vi "Format CSV.vi"(8 "error in (no error)":errorcluster, 9 "delimiter":string=",", 10 "CSV File Input":path, 11 "Original CSV Format":enum16{"Format A", "Format B"}(ring)) -> (0 "error out":errorcluster, 1 "Parcel Length":i32[](array[numeric]), 2 "All Terminal Data":T1(array[cluster]))   [LabVIEW 2017] (continued)
"22:36.1", "22:36.1", "22:36.2", "22:36.2", "22:36.2", "22:36.3", "22:36.3", "22:36.3", "22:36.4", "22:36.4", "22:36.4", "22:36.5", "22:36.5", "22:36.5", "22:36.6", "22:36.6", "22:36.6", "22:36.7", "22:36.7", "22:36.7", "22:36.8", "22:36.8", "22:36.8", "22:36.9", "22:36.9", "22:36.9", "22:37.0", "22:37.0", "22:37.0", "22:37.1", "22:37.1", "22:37.1", "22:37.2", "22:37.2", "22:37.2", "22:37.3", "22:37.3", "22:37.3", "22:37.4", "22:37.4", "22:37.4", "22:37.5", "22:37.5", "22:37.5", "22:37.6", "22:37.6", "22:37.6", "22:37.7", "22:37.7", "22:37.7", "22:37.8", "22:37.8", "22:37.8", "22:37.9", "22:37.9", "22:37.9", "22:38.0", "22:38.0", "22:38.0", "22:38.1", "22:38.1", "22:38.1", "22:38.2", "22:38.2", "22:38.2", "22:38.3", "22:38.3", "22:38.3", "22:38.4", "22:38.4", "22:38.4", "22:38.5", "22:38.5", "22:38.5", "22:38.6", "22:38.6", "22:38.6", "22:38.7", "22:38.7", "22:38.7", "22:38.8", "22:38.8", "22:38.8", "22:38.9", "22:38.9", "22:38.9", "22:39.0", "22:39.0", "22:39.0", "22:39.1", "22:39.1", "22:39.1", "22:39.2", "22:39.2", "22:39.2", "22:39.3", "22:39.3", "22:39.3", "22:39.4", "22:39.4", "22:39.4", "22:39.5", "22:39.5", "22:39.5", "22:39.6", "22:39.6", "22:39.6", "22:39.7", "22:39.7", "22:39.7", "22:39.8", "22:39.8", "22:39.8", "22:39.9", "22:39.9", "22:39.9", "22:40.0", "22:40.0", "22:40.0", "22:40.1", "22:40.1", "22:40.1", "22:40.2", "22:40.2", "22:40.2", "22:40.3", "22:40.3", "22:40.3", "22:40.4", "22:40.4", "22:40.4", "22:40.5", "22:40.5", "22:40.5", "22:40.6", "22:40.6", "22:40.6", "22:40.7", "22:40.7", "22:40.7", "22:40.8", "22:40.8", "22:40.8", "22:40.9", "22:40.9", "22:40.9", "22:41.0", "22:41.0", "22:41.0", "22:41.1", "22:41.1", "22:41.1", "22:41.2", "22:41.2", "22:41.2", "22:41.3", "22:41.3", "22:41.3", "22:41.4", "22:41.4", "22:41.4", "22:41.5", "22:41.5", "22:41.5", "22:41.6", "22:41.6", "22:41.6", "22:41.7", "22:41.7", "22:41.7", "22:41.8", "22:41.8", "22:41.8", "22:41.9", "22:41.9", "22:41.9", "22:42.0", "22:42.0", "22:42.0", "22:42.1", "22:42.1", "22:42.1", "22:42.2", "22:42.2", "22:42.2", "22:42.3", "22:42.3", "22:42.3", "22:42.4", "22:42.4", "22:42.4", "22:42.5", "22:42.5", "22:42.5", "22:42.6", "22:42.6", "22:42.6", "22:42.7", "22:42.7", "22:42.7", "22:42.8", "22:42.8", "22:42.8", "22:42.9", "22:42.9", "22:42.9", "22:43.0", "22:43.0", "22:43.0", "22:43.1", "22:43.1", "22:43.1", "22:43.2", "22:43.2", "22:43.2", "22:43.3", "22:43.3", "22:43.3", "22:43.4", "22:43.4", "22:43.4", "22:43.5", "22:43.5", "22:43.5", "22:43.6", "22:43.6", "22:43.6", "22:43.7", "22:43.7", "22:43.7", "22:43.8", "22:43.8", "22:43.8", "22:43.9", "22:43.9", "22:43.9", "22:44.0", "22:44.0", "22:44.0", "22:44.1", "22:44.1", "22:44.1", "22:44.2", "22:44.2", "22:44.2", "22:44.3", "22:44.3", "22:44.3", "22:44.4", "22:44.4", "22:44.4", "22:44.5", "22:44.5", "22:44.5", "22:44.6", "22:44.6", "22:44.6", "22:44.7", "22:44.7", "22:44.7", "22:44.8", "22:44.8", "22:44.8", "22:44.9", "22:44.9", "22:44.9", "22:45.0", "22:45.0", "22:45.0", "22:45.1", "22:45.1", "22:45.1", "22:45.2", "22:45.2", "22:45.2", "22:45.3", "22:45.3", "22:45.3", "22:45.4", "22:45.4", "22:45.4", "22:45.5", "22:45.5", "22:45.5", "22:45.6", "22:45.6", "22:45.6", "22:45.7", "22:45.7", "22:45.7", "22:45.8", "22:45.8", "22:45.8", "22:45.9", "22:45.9", "22:45.9", "22:46.0", "22:46.0", "22:46.0", "22:46.1", "22:46.1", "22:46.1", "22:46.2", "22:46.2", "22:46.2", "22:46.3", "22:46.3", "22:46.3", "22:46.4", "22:46.4", "22:46.4", "22:46.5", "22:46.5", "22:46.5", "22:46.6", "22:46.6", "22:46.6", "22:46.7", "22:46.7", "22:46.7", "22:46.8", "22:46.8", "22:46.8", "22:46.9", "22:46.9", "22:46.9", "22:47.0", "22:47.0", "22:47.0", "22:47.1", "22:47.1", "22:47.1", "22:47.2", "22:47.2", "22:47.2", "22:47.3", "22:47.3", "22:47.3", "22:47.4", "22:47.4", "22:47.4", "22:47.5", "22:47.5", "22:47.5", "22:47.6", "22:47.6", "22:47.6", "22:47.7", "22:47.7", "22:47.7", "22:47.8", "22:47.8", "22:47.8", "22:47.9", "22:47.9", "22:47.9", "22:48.0", "22:48.0", "22:48.0", "22:48.1", "22:48.1", "22:48.1", "22:48.2", "22:48.2", "22:48.2", "22:48.3", "22:48.3", "22:48.3", "22:48.4", "22:48.4", "22:48.4", "22:48.5", "22:48.5", "22:48.5", "22:48.6", "22:48.6", "22:48.6", "22:48.7", "22:48.7", "22:48.7", "22:48.8", "22:48.8", "22:48.8", "22:48.9", "22:48.9", "22:48.9", "22:49.0", "22:49.0", "22:49.0", "22:49.1", "22:49.1", "22:49.1", "22:49.2", "22:49.2", "22:49.2", "22:49.3", "22:49.3", "22:49.3", "22:49.4", "22:49.4", "22:49.4", "22:49.5", "22:49.5", "22:49.5", "22:49.6", "22:49.6", "22:49.6", "22:49.7", "22:49.7", "22:49.7", "22:49.8", "22:49.8", "22:49.8", "22:49.9", "22:49.9", "22:49.9", "22:50.0", "22:50.0", "22:50.0", "22:50.1", "22:50.1", "22:50.1", "22:50.2", "22:50.2", "22:50.2", "22:50.3", "22:50.3", "22:50.3", "22:50.4", "22:50.4", "22:50.4", "22:50.5", "22:50.5", "22:50.5", "22:50.6", "22:50.6", "22:50.6", "22:50.7", "22:50.7", "22:50.7", "22:50.8", "22:50.8", "22:50.8", "22:50.9", "22:50.9", "22:50.9", "22:51.0", "22:51.0", "22:51.0", "22:51.1", "22:51.1", "22:51.1", "22:51.2", "22:51.2", "22:51.2", "22:51.3", "22:51.3", "22:51.3", "22:51.4", "22:51.4", "22:51.4", "22:51.5", "22:51.5", "22:51.5", "22:51.6", "22:51.6", "22:51.6", "22:51.7", "22:51.7", "22:51.7", "22:51.8", "22:51.8", "22:51.8", "22:51.9", "22:51.9", "22:51.9", "22:52.0", "22:52.0", "22:52.0", "22:52.1", "22:52.1", "22:52.1", "22:52.2", "22:52.2", "22:52.2", "22:52.3", "22:52.3", "22:52.3", "22:52.4", "22:52.4", "22:52.4", "22:52.5", "22:52.5", "22:52.5", "22:52.6", "22:52.6", "22:52.6", "22:52.7", "22:52.7", "22:52.7", "22:52.8", "22:52.8", "22:52.8", "22:52.9", "22:52.9", "22:52.9", "22:53.0", "22:53.0", "22:53.0", "22:53.1", "22:53.1", "22:53.1", "22:53.2", "22:53.2", "22:53.2", "22:53.3", "22:53.3", "22:53.3", "22:53.4", "22:53.4", "22:53.4", "22:53.5", "22:53.5", "22:53.5", "22:53.6", "22:53.6", "22:53.6", "22:53.7", "22:53.7", "22:53.7", "22:53.8", "22:53.8", "22:53.8", "22:53.9", "22:53.9", "22:53.9", "22:54.0", "22:54.0", "22:54.0", "22:54.1", "22:54.1", "22:54.1", "22:54.2", "22:54.2", "22:54.2", "22:54.3", "22:54.3", "22:54.3", "22:54.4", "22:54.4", "22:54.4", "22:54.5", "22:54.5", "22:54.5", "22:54.6", "22:54.6", "22:54.6", "22:54.7", "22:54.7", "22:54.7", "22:54.8", "22:54.8", "22:54.8", "22:54.9", "22:54.9", "22:54.9", "22:55.0", "22:55.0", "22:55.0", "22:55.1", "22:55.1", "22:55.1", "22:55.2", "22:55.2", "22:55.2", "22:55.3", "22:55.3", "22:55.3", "22:55.4", "22:55.4", "22:55.4", "22:55.5", "22:55.5", "22:55.5", "22:55.6", "22:55.6", "22:55.6", "22:55.7", "22:55.7", "22:55.7", "22:55.8", "22:55.8", "22:55.8", "22:55.9", "22:55.9", "22:55.9", "22:56.0", "22:56.0", "22:56.0", "22:56.1", "22:56.1", "22:56.1", "22:56.2", "22:56.2", "22:56.2", "22:56.3", "22:56.3", "22:56.3", "22:56.4", "22:56.4", "22:56.4", "22:56.5", "22:56.5", "22:56.5", "22:56.6", "22:56.6", "22:56.6", "22:56.7", "22:56.7", "22:56.7", "22:56.8", "22:56.8", "22:56.8", "22:56.9", "22:56.9", "22:56.9", "22:57.0", "22:57.0", "22:57.0", "22:57.1", "22:57.1", "22:57.1", "22:57.2", "22:57.2", "22:57.2", "22:57.3", "22:57.3", "22:57.3", "22:57.4", "22:57.4", "22:57.4", "22:57.5", "22:57.5", "22:57.5", "22:57.6", "22:57.6", "22:57.6", "22:57.7", "22:57.7", "22:57.7", "22:57.8", "22:57.8", "22:57.8", "22:57.9", "22:57.9", "22:57.9", "22:58.0", "22:58.0", "22:58.0", "22:58.1", "22:58.1", "22:58.1", "22:58.2", "22:58.2", "22:58.2", "22:58.3", "22:58.3", "22:58.3", "22:58.4", "22:58.4", "22:58.4", "22:58.5", "22:58.5", "22:58.5", "22:58.6", "22:58.6", "22:58.6", "22:58.7", "22:58.7", "22:58.7", "22:58.8", "22:58.8", "22:58.8", "22:58.9", "22:58.9", "22:58.9", "22:59.0", "22:59.0", "22:59.0", "22:59.1", "22:59.1", "22:59.1", "22:59.2", "22:59.2", "22:59.2", "22:59.3", "22:59.3", "22:59.3", "22:59.4", "22:59.4", "22:59.4", "22:59.5", "22:59.5", "22:59.5", "22:59.6", "22:59.6", "22:59.6", "22:59.7", "22:59.7", "22:59.7", "22:59.8", "22:59.8", "22:59.8", "22:59.9", "22:59.9", "22:59.9", "23:00.0", "23:00.0", "23:00.0", "23:00.1", "23:00.1", "23:00.1", "23:00.2", "23:00.2", "23:00.2", "23:00.3", "23:00.3", "23:00.3", "23:00.4", "23:00.4", "23:00.4", "23:00.5", "23:00.5", "23:00.5", "23:00.6", "23:00.6", "23:00.6", "23:00.7", "23:00.7", "23:00.7", "23:00.8", "23:00.8", "23:00.8", "23:00.9", "23:00.9", "23:00.9", "23:01.0", "23:01.0", "23:01.0", "23:01.1", "23:01.1", "23:01.1", "23:01.2", "23:01.2", "23:01.2", "23:01.3", "23:01.3", "23:01.3", "23:01.4", "23:01.4", "23:01.4", "23:01.5", "23:01.5", "23:01.5", "23:01.6", "23:01.6", "23:01.6", "23:01.7", "23:01.7", "23:01.7", "23:01.8", "23:01.8", "23:01.8", "23:01.9", "23:01.9", "23:01.9", "23:02.0", "23:02.0", "23:02.0", "23:02.1", "23:02.1", "23:02.1", "23:02.2", "23:02.2", "23:02.2", "23:02.3", "23:02.3", "23:02.3", "23:02.4", "23:02.4", "23:02.4", "23:02.5", "23:02.5", "23:02.5", "23:02.6", "23:02.6", "23:02.6", "23:02.7", "23:02.7", "23:02.7", "23:02.8", "23:02.8", "23:02.8", "23:02.9", "23:02.9", "23:02.9", "23:03.0", "23:03.0", "23:03.0", "23:03.1", "23:03.1", "23:03.1", "23:03.2", "23:03.2", "23:03.2", "23:03.3", "23:03.3", "23:03.3", "23:03.4", "23:03.4", "23:03.4", "23:03.5", "23:03.5", "23:03.5", "23:03.6", "23:03.6", "23:03.6", "23:03.7", "23:03.7", "23:03.7", "23:03.8", "23:03.8", "23:03.8", "23:03.9", "23:03.9", "23:03.9", "23:04.0", "23:04.0", "23:04.0", "23:04.1", "23:04.1", "23:04.1", "23:04.2", "23:04.2", "23:04.2", "23:04.3", "23:04.3", "23:04.3", "23:04.4", "23:04.4", "23:04.4", "23:04.5", "23:04.5", "23:04.5", "23:04.6", "23:04.6", "23:04.6", "23:04.7", "23:04.7", "23:04.7", "23:04.8", "23:04.8", "23:04.8", "23:04.9", "23:04.9", "23:04.9", "23:05.0", "23:05.0", "23:05.0", "23:05.1", "23:05.1", "23:05.1", "23:05.2", "23:05.2", "23:05.2", "23:05.3", "23:05.3", "23:05.3", "23:05.4", "23:05.4", "23:05.4", "23:05.5", "23:05.5", "23:05.5", "23:05.6", "23:05.6", "23:05.6", "23:05.7", "23:05.7", "23:05.7", "23:05.8", "23:05.8", "23:05.8", "23:05.9", "23:05.9", "23:05.9", "23:06.0", "23:06.0", "23:06.0", "23:06.1", "23:06.1", "23:06.1", "23:06.2", "23:06.2", "23:06.2", "23:06.3", "23:06.3", "23:06.3", "23:06.4", "23:06.4", "23:06.4", "23:06.5", "23:06.5", "23:06.5", "23:06.6", "23:06.6", "23:06.6", "23:06.7", "23:06.7", "23:06.7", "23:06.8", "23:06.8", "23:06.8", "23:06.9", "23:06.9", "23:06.9", "23:07.0", "23:07.0", "23:07.0", "23:07.1", "23:07.1", "23:07.1", "23:07.2", "23:07.2", "23:07.2", "23:07.3", "23:07.3", "23:07.3", "23:07.4", "23:07.4", "23:07.4", "23:07.5", "23:07.5", "23:07.5", "23:07.6", "23:07.6", "23:07.6", "23:07.7", "23:07.7", "23:07.7", "23:07.8", "23:07.8", "23:07.8", "23:07.9", "23:07.9", "23:07.9", "23:08.0", "23:08.0", "23:08.0", "23:08.1", "23:08.1", "23:08.1", "23:08.2", "23:08.2", "23:08.2", "23:08.3", "23:08.3", "23:08.3", "23:08.4", "23:08.4", "23:08.4", "23:08.5", "23:08.5", "23:08.5", "23:08.6", "23:08.6", "23:08.6", "23:08.7", "23:08.7", "23:08.7", "23:08.8", "23:08.8", "23:08.8", "23:08.9", "23:08.9", "23:08.9", "23:09.0", "23:09.0", "23:09.0", "23:09.1", "23:09.1", "23:09.1", "23:09.2", "23:09.2", "23:09.2", "23:09.3", "23:09.3", "23:09.3", "23:09.4", "23:09.4", "23:09.4", "23:09.5", "23:09.5", "23:09.5", "23:09.6", "23:09.6", "23:09.6", "23:09.7", "23:09.7", "23:09.7", "23:09.8", "23:09.8", "23:09.8", "23:09.9", "23:09.9", "23:09.9", "23:10.0", "23:10.0", "23:10.0", "23:10.1", "23:10.1", "23:10.1", "23:10.2", "23:10.2", "23:10.2", "23:10.3", "23:10.3", "23:10.3", "23:10.4", "23:10.4", "23:10.4", "23:10.5", "23:10.5", "23:10.5", "23:10.6", "23:10.6", "23:10.6", "23:10.7", "23:10.7", "23:10.7", "23:10.8", "23:10.8", "23:10.8", "23:10.9", "23:10.9", "23:10.9", "23:11.0", "23:11.0", "23:11.0", "23:11.1", "23:11.1", "23:11.1", "23:11.2", "23:11.2", "23:11.2", "23:11.3", "23:11.3", "23:11.3", "23:11.4", "23:11.4", "23:11.4", "23:11.5", "23:11.5", "23:11.5", "23:11.6", "23:11.6", "23:11.6", "23:11.7", "23:11.7", "23:11.7", "23:11.8", "23:11.8", "23:11.8", "23:11.9", "23:11.9", "23:11.9", "23:12.0", "23:12.0", "23:12.0", "23:12.1", "23:12.1", "23:12.1", "23:12.2", "23:12.2", "23:12.2", "23:12.3", "23:12.3", "23:12.3", "23:12.4", "23:12.4", "23:12.4", "23:12.5", "23:12.5", "23:12.5", "23:12.6", "23:12.6", "23:12.6", "23:12.7", "23:12.7", "23:12.7", "23:12.8", "23:12.8", "23:12.8", "23:12.9", "23:12.9", "23:12.9", "23:13.0", "23:13.0", "23:13.0", "23:13.1", "23:13.1", "23:13.1", "23:13.2", "23:13.2", "23:13.2", "23:13.3", "23:13.3", "23:13.3", "23:13.4", "23:13.4", "23:13.4", "23:13.5", "23:13.5", "23:13.5", "23:13.6", "23:13.6", "23:13.6", "23:13.7", "23:13.7", "23:13.7", "23:13.8", "23:13.8", "23:13.8", "23:13.9", "23:13.9", "23:13.9", "23:14.0", "23:14.0", "23:14.0", "23:14.1", "23:14.1", "23:14.1", "23:14.2", "23:14.2", "23:14.2", "23:14.3", "23:14.3", "23:14.3", "23:14.4", "23:14.4", "23:14.4", "23:14.5", "23:14.5", "23:14.5", "23:14.6", "23:14.6", "23:14.6", "23:14.7", "23:14.7", "23:14.7", "23:14.8", "23:14.8", "23:14.8", "23:14.9", "23:14.9", "23:14.9", "23:15.0", "23:15.0", "23:15.0", "23:15.1", "23:15.1", "23:15.1", "23:15.2", "23:15.2", "23:15.2", "23:15.3", "23:15.3", "23:15.3", "23:15.4", "23:15.4", "23:15.4", "23:15.5", "23:15.5", "23:15.5", "23:15.6", "23:15.6", "23:15.6", "23:15.7", "23:15.7", "23:15.7", "23:15.8", "23:15.8", "23:15.8", "23:15.9", "23:15.9", "23:15.9", "23:16.0", "23:16.0", "23:16.0", "23:16.1", "23:16.1", "23:16.1", "23:16.2", "23:16.2", "23:16.2", "23:16.3", "23:16.3", "23:16.3", "23:16.4", "23:16.4", "23:16.4", "23:16.5", "23:16.5", "23:16.5", "23:16.6", "23:16.6", "23:16.6", "23:16.7", "23:16.7", "23:16.7", "23:16.8", "23:16.8", "23:16.8", "23:16.9", "23:16.9", "23:16.9", "23:17.0", "23:17.0", "23:17.0", "23:17.1", "23:17.1", "23:17.1", "23:17.2", "23:17.2", "23:17.2", "23:17.3", "23:17.3", "23:17.3", "23:17.4", "23:17.4", "23:17.4", "23:17.5", "23:17.5", "23:17.5", "23:17.6", "23:17.6", "23:17.6", "23:17.7", "23:17.7", "23:17.7", "23:17.8", "23:17.8", "23:17.8", "23:17.9", "23:17.9", "23:17.9", "23:18.0", "23:18.0", "23:18.0", "23:18.1", "23:18.1", "23:18.1", "23:18.2", "23:18.2", "23:18.2", "23:18.3", "23:18.3", "23:18.3", "23:18.4", "23:18.4", "23:18.4", "23:18.5", "23:18.5", "23:18.5", "23:18.6", "23:18.6", "23:18.6", "23:18.7", "23:18.7", "23:18.7", "23:18.8", "23:18.8", "23:18.8", "23:18.9", "23:18.9", "23:18.9", "23:19.0", "23:19.0", "23:19.0", "23:19.1", "23:19.1", "23:19.1", "23:19.2", "23:19.2", "23:19.2", "23:19.3", "23:19.3", "23:19.3", "23:19.4", "23:19.4", "23:19.4", "23:19.5", "23:19.5", "23:19.5", "23:19.6", "23:19.6", "23:19.6", "23:19.7", "23:19.7", "23:19.7", "23:19.8", "23:19.8", "23:19.8", "23:19.9", "23:19.9", "23:19.9", "23:20.0", "23:20.0", "23:20.0", "23:20.1", "23:20.1", "23:20.1", "23:20.2", "23:20.2", "23:20.2", "23:20.3", "23:20.3", "23:20.3", "23:20.4", "23:20.4", "23:20.4", "23:20.5", "23:20.5", "23:20.5", "23:20.6", "23:20.6", "23:20.6", "23:20.7", "23:20.7", "23:20.7", "23:20.8", "23:20.8", "23:20.8", "23:20.9", "23:20.9", "23:20.9", "23:21.0", "23:21.0", "23:21.0", "23:21.1", "23:21.1", "23:21.1", "23:21.2", "23:21.2", "23:21.2", "23:21.3", "23:21.3", "23:21.3", "23:21.4", "23:21.4", "23:21.4", "23:21.5", "23:21.5", "23:21.5", "23:21.6", "23:21.6", "23:21.6", "23:21.7", "23:21.7", "23:21.7", "23:21.8", "23:21.8", "23:21.8", "23:21.9", "23:21.9", "23:21.9", "23:22.0", "23:22.0", "23:22.0", "23:22.1", "23:22.1", "23:22.1", "23:22.2", "23:22.2", "23:22.2", "23:22.3", "23:22.3", "23:22.3", "23:22.4", "23:22.4", "23:22.4", "23:22.5", "23:22.5", "23:22.5", "23:22.6", "23:22.6", "23:22.6", "23:22.7", "23:22.7", "23:22.7", "23:22.8", "23:22.8", "23:22.8", "23:22.9", "23:22.9", "23:22.9", "23:23.0", "23:23.0", "23:23.0", "23:23.1", "23:23.1", "23:23.1", "23:23.2", "23:23.2", "23:23.2", "23:23.3", "23:23.3", "23:23.3", "23:23.4", "23:23.4", "23:23.4", "23:23.5", "23:23.5", "23:23.5", "23:23.6", "23:23.6", "23:23.6", "23:23.7", "23:23.7", "23:23.7", "23:23.8", "23:23.8", "23:23.8", "23:23.9", "23:23.9", "23:23.9", "23:24.0", "23:24.0", "23:24.0", "23:24.1", "23:24.1", "23:24.1", "23:24.2", "23:24.2", "23:24.2", "23:24.3", "23:24.3", "23:24.3", "23:24.4", "23:24.4", "23:24.4", "23:24.5", "23:24.5", "23:24.5", "23:24.6", "23:24.6", "23:24.6", "23:24.7", "23:24.7", "23:24.7", "23:24.8", "23:24.8", "23:24.8", "23:24.9", "23:24.9", "23:24.9", "23:25.0", "23:25.0", "23:25.0", "23:25.1", "23:25.1", "23:25.1", "23:25.2", "23:25.2", "23:25.2", "23:25.3", "23:25.3", "23:25.3", "23:25.4", "23:25.4", "23:25.4", "23:25.5", "23:25.5", "23:25.5", "23:25.6", "23:25.6", "23:25.6", "23:25.7", "23:25.7", "23:25.7", "23:25.8", "23:25.8", "23:25.8", "23:25.9", "23:25.9", "23:25.9", "23:26.0", "23:26.0", "23:26.0", "23:26.1", "23:26.1", "23:26.1", "23:26.2", "23:26.2", "23:26.2", "23:26.3", "23:26.3", "23:26.3", "23:26.4", "23:26.4", "23:26.4", "23:26.5", "23:26.5", "23:26.5", "23:26.6", "23:26.6", "23:26.6", "23:26.7", "23:26.7", "23:26.7", "23:26.8", "23:26.8", "23:26.8", "23:26.9", "23:26.9", "23:26.9", "23:27.0", "23:27.0", "23:27.0", "23:27.1", "23:27.1", "23:27.1", "23:27.2", "23:27.2", "23:27.2", "23:27.3", "23:27.3", "23:27.3", "23:27.4", "23:27.4", "23:27.4", "23:27.5", "23:27.5", "23:27.5", "23:27.6", "23:27.6", "23:27.6", "23:27.7", "23:27.7", "23:27.7", "23:27.8", "23:27.8", "23:27.8", "23:27.9", "23:27.9", "23:27.9", "23:28.0", "23:28.0", "23:28.0", "23:28.1", "23:28.1", "23:28.1", "23:28.2", "23:28.2", "23:28.2", "23:28.3", "23:28.3", "23:28.3", "23:28.4", "23:28.4", "23:28.4", "23:28.5", "23:28.5", "23:28.5", "23:28.6", "23:28.6", "23:28.6", "23:28.7", "23:28.7", "23:28.7", "23:28.8", "23:28.8", "23:28.8", "23:28.9", "23:28.9", "23:28.9", "23:29.0", "23:29.0", "23:29.0", "23:29.1", "23:29.1", "23:29.1", "23:29.2", "23:29.2", "23:29.2", "23:29.3", "23:29.3", "23:29.3", "23:29.4", "23:29.4", "23:29.4", "23:29.5", "23:29.5", "23:29.5", "23:29.6", "23:29.6", "23:29.6", "23:29.7", "23:29.7", "23:29.7", "23:29.8", "23:29.8", "23:29.8", "23:29.9", "23:29.9", "23:29.9", "23:30.0", "23:30.0", "23:30.0", "23:30.1", "23:30.1", "23:30.1", "23:30.2", "23:30.2", "23:30.2", "23:30.3", "23:30.3", "23:30.3", "23:30.4", "23:30.4", "23:30.4", "23:30.5", "23:30.5", "23:30.5", "23:30.6", "23:30.6", "23:30.6", "23:30.7", "23:30.7", "23:30.7", "23:30.8", "23:30.8", "23:30.8", "23:30.9", "23:30.9", "23:30.9", "23:31.0", "23:31.0", "23:31.0", "23:31.1", "23:31.1", "23:31.1", "23:31.2", "23:31.2", "23:31.2", "23:31.3", "23:31.3", "23:31.3", "23:31.4", "23:31.4", "23:31.4", "23:31.5", "23:31.5", "23:31.5", "23:31.6", "23:31.6", "23:31.6", "23:31.7", "23:31.7", "23:31.7", "23:31.8", "23:31.8", "23:31.8", "23:31.9", "23:31.9", "23:31.9", "23:32.0", "23:32.0", "23:32.0", "23:32.1", "23:32.1", "23:32.1", "23:32.2", "23:32.2", "23:32.2", "23:32.3", "23:32.3", "23:32.3", "23:32.4", "23:32.4", "23:32.4", "23:32.5", "23:32.5", "23:32.5", "23:32.6", "23:32.6", "23:32.6", "23:32.7", "23:32.7", "23:32.7", "23:32.8", "23:32.8", "23:32.8", "23:32.9", "23:32.9", "23:32.9", "23:33.0", "23:33.0", "23:33.0", "23:33.1", "23:33.1", "23:33.1", "23:33.2", "23:33.2", "23:33.2", "23:33.3", "23:33.3", "23:33.3", "23:33.4", "23:33.4", "23:33.4", "23:33.5", "23:33.5", "23:33.5", "23:33.6", "23:33.6", "23:33.6", "23:33.7", "23:33.7", "23:33.7", "23:33.8", "23:33.8", "23:33.8", "23:33.9", "23:33.9", "23:33.9", "23:34.0", "23:34.0", "23:34.0", "23:34.1", "23:34.1", "23:34.1", "23:34.2", "23:34.2", "23:34.2", "23:34.3", "23:34.3", "23:34.3", "23:34.4", "23:34.4", "23:34.4", "23:34.5", "23:34.5", "23:34.5", "23:34.6", "23:34.6", "23:34.6", "23:34.7", "23:34.7", "23:34.7", "23:34.8", "23:34.8", "23:34.8", "23:34.9", "23:34.9", "23:34.9", "23:35.0", "23:35.0", "23:35.0", "23:35.1", "23:35.1", "23:35.1", "23:35.2", "23:35.2", "23:35.2", "23:35.3", "23:35.3", "23:35.3", "23:35.4", "23:35.4", "23:35.4", "23:35.5", "23:35.5", "23:35.5", "23:35.6", "23:35.6", "23:35.6", "23:35.7", "23:35.7", "23:35.7", "23:35.8", "23:35.8", "23:35.8", "23:35.9", "23:35.9", "23:35.9", "23:36.0", "23:36.0", "23:36.0", "23:36.1", "23:36.1", "23:36.1", "23:36.2", "23:36.2", "23:36.2", "23:36.3", "23:36.3", "23:36.3", "23:36.4", "23:36.4", "23:36.4", "23:36.5", "23:36.5", "23:36.5", "23:36.6", "23:36.6", "23:36.6", "23:36.7", "23:36.7", "23:36.7", "23:36.8", "23:36.8", "23:36.8", "23:36.9", "23:36.9", "23:36.9", "23:37.0", "23:37.0", "23:37.0", "23:37.1", "23:37.1", "23:37.1", "23:37.2", "23:37.2", "23:37.2", "23:37.3", "23:37.3", "23:37.3", "23:37.4", "23:37.4", "23:37.4", "23:37.5", "23:37.5", "23:37.5", "23:37.6", "23:37.6", "23:37.6", "23:37.7", "23:37.7", "23:37.7", "23:37.8", "23:37.8", "23:37.8", "23:37.9", "23:37.9", "23:37.9", "23:38.0", "23:38.0", "23:38.0", "23:38.1", "23:38.1", "23:38.1", "23:38.2", "23:38.2", "23:38.2", "23:38.3", "23:38.3", "23:38.3", "23:38.4", "23:38.4", "23:38.4", "23:38.5", "23:38.5", "23:38.5", "23:38.6", "23:38.6", "23:38.6", "23:38.7", "23:38.7", "23:38.7", "23:38.8", "23:38.8", "23:38.8", "23:38.9", "23:38.9", "23:38.9", "23:39.0", "23:39.0", "23:39.0", "23:39.1", "23:39.1", "23:39.1", "23:39.2", "23:39.2", "23:39.2", "23:39.3", "23:39.3", "23:39.3", "23:39.4", "23:39.4", "23:39.4", "23:39.5", "23:39.5", "23:39.5", "23:39.6", "23:39.6", "23:39.6", "23:39.7", "23:39.7", "23:39.7", "23:39.8", "23:39.8", "23:39.8", "23:39.9", "23:39.9", "23:39.9", "23:40.0", "23:40.0", "23:40.0", "23:40.1", "23:40.1", "23:40.1", "23:40.2", "23:40.2", "23:40.2", "23:40.3", "23:40.3", "23:40.3", "23:40.4", "23:40.4", "23:40.4", "23:40.5", "23:40.5", "23:40.5", "23:40.6", "23:40.6", "23:40.6", "23:40.7", "23:40.7", "23:40.7", "23:40.8", "23:40.8", "23:40.8", "23:40.9", "23:40.9", "23:40.9", "23:41.0", "23:41.0", "23:41.0", "23:41.1", "23:41.1", "23:41.1", "23:41.2", "23:41.2", "23:41.2", "23:41.3", "23:41.3", "23:41.3", "23:41.4", "23:41.4", "23:41.4", "23:41.5", "23:41.5", "23:41.5", "23:41.6", "23:41.6", "23:41.6", "23:41.7", "23:41.7", "23:41.7", "23:41.8", "23:41.8", "23:41.8", "23:41.9", "23:41.9", "23:41.9", "23:42.0", "23:42.0", "23:42.0", "23:42.1", "23:42.1", "23:42.1", "23:42.2", "23:42.2", "23:42.2", "23:42.3", "23:42.3", "23:42.3", "23:42.4", "23:42.4", "23:42.4", "23:42.5", "23:42.5", "23:42.5", "23:42.6", "23:42.6", "23:42.6", "23:42.7", "23:42.7", "23:42.7", "23:42.8", "23:42.8", "23:42.8", "23:42.9", "23:42.9", "23:42.9", "23:43.0", "23:43.0", "23:43.0", "23:43.1", "23:43.1", "23:43.1", "23:43.2", "23:43.2", "23:43.2", "23:43.3", "23:43.3", "23:43.3", "23:43.4", "23:43.4", "23:43.4", "23:43.5", "23:43.5", "23:43.5", "23:43.6", "23:43.6", "23:43.6", "23:43.7", "23:43.7", "23:43.7", "23:43.8", "23:43.8", "23:43.8", "23:43.9", "23:43.9", "23:43.9", "23:44.0", "23:44.0", "23:44.0", "23:44.1", "23:44.1", "23:44.1", "23:44.2", "23:44.2", "23:44.2", "23:44.3", "23:44.3", "23:44.3", "23:44.4", "23:44.4", "23:44.4", "23:44.5", "23:44.5", "23:44.5", "23:44.6", "23:44.6", "23:44.6", "23:44.7", "23:44.7", "23:44.7", "23:44.8", "23:44.8", "23:44.8", "23:44.9", "23:44.9", "23:44.9", "23:45.0", "23:45.0", "23:45.0", "23:45.1", "23:45.1", "23:45.1", "23:45.2", "23:45.2", "23:45.2", "23:45.3", "23:45.3", "23:45.3", "23:45.4", "23:45.4", "23:45.4", "23:45.5", "23:45.5", "23:45.5", "23:45.6", "23:45.6", "23:45.6", "23:45.7", "23:45.7", "23:45.7", "23:45.8", "23:45.8", "23:45.8", "23:45.9", "23:45.9", "23:45.9", "23:46.0", "23:46.0", "23:46.0", "23:46.1", "23:46.1", "23:46.1", "23:46.2", "23:46.2", "23:46.2", "23:46.3", "23:46.3", "23:46.3", "23:46.4", "23:46.4", "23:46.4", "23:46.5", "23:46.5", "23:46.5", "23:46.6", "23:46.6", "23:46.6", "23:46.7", "23:46.7", "23:46.7", "23:46.8", "23:46.8", "23:46.8", "23:46.9", "23:46.9", "23:46.9", "23:47.0", "23:47.0", "23:47.0", "23:47.1", "23:47.1", "23:47.1", "23:47.2", "23:47.2", "23:47.2", "23:47.3", "23:47.3", "23:47.3", "23:47.4", "23:47.4", "23:47.4", "23:47.5", "23:47.5", "23:47.5", "23:47.6", "23:47.6", "23:47.6", "23:47.7", "23:47.7", "23:47.7", "23:47.8", "23:47.8", "23:47.8", "23:47.9", "23:47.9", "23:47.9", "23:48.0", "23:48.0", "23:48.0", "23:48.1", "23:48.1", "23:48.1", "23:48.2", "23:48.2", "23:48.2", "23:48.3", "23:48.3", "23:48.3", "23:48.4", "23:48.4", "23:48.4", "23:48.5", "23:48.5", "23:48.5", "23:48.6", "23:48.6", "23:48.6", "23:48.7", "23:48.7", "23:48.7", "23:48.8", "23:48.8", "23:48.8", "23:48.9", "23:48.9", "23:48.9", "23:49.0", "23:49.0", "23:49.0", "23:49.1", "23:49.1", "23:49.1", "23:49.2", "23:49.2", "23:49.2", "23:49.3", "23:49.3", "23:49.3", "23:49.4", "23:49.4", "23:49.4", "23:49.5", "23:49.5", "23:49.5", "23:49.6", "23:49.6", "23:49.6", "23:49.7", "23:49.7", "23:49.7", "23:49.8", "23:49.8", "23:49.8", "23:49.9", "23:49.9", "23:49.9", "23:50.0", "23:50.0", "23:50.0", "23:50.1", "23:50.1", "23:50.1", "23:50.2", "23:50.2", "23:50.2", "23:50.3", "23:50.3", "23:50.3", "23:50.4", "23:50.4", "23:50.4", "23:50.5", "23:50.5", "23:50.5", "23:50.6", "23:50.6", "23:50.6", "23:50.7", "23:50.7", "23:50.7", "23:50.8", "23:50.8", "23:50.8", "23:50.9", "23:50.9", "23:50.9", "23:51.0", "23:51.0", "23:51.0", "23:51.1", "23:51.1", "23:51.1", "23:51.2", "23:51.2", "23:51.2", "23:51.3", "23:51.3", "23:51.3", "23:51.4", "23:51.4", "23:51.4", "23:51.5", "23:51.5", "23:51.5", "23:51.6", "23:51.6", "23:51.6", "23:51.7", "23:51.7", "23:51.7", "23:51.8", "23:51.8", "23:51.8", "23:51.9", "23:51.9", "23:51.9", "23:52.0", "23:52.0", "23:52.0", "23:52.1", "23:52.1", "23:52.1", "23:52.2", "23:52.2", "23:52.2", "23:52.3", "23:52.3", "23:52.3", "23:52.4", "23:52.4", "23:52.4", "23:52.5", "23:52.5", "23:52.5", "23:52.6", "23:52.6", "23:52.6", "23:52.7", "23:52.7", "23:52.7", "23:52.8", "23:52.8", "23:52.8", "23:52.9", "23:52.9", "23:52.9", "23:53.0", "23:53.0", "23:53.0", "23:53.1", "23:53.1", "23:53.1", "23:53.2", "23:53.2", "23:53.2", "23:53.3", "23:53.3", "23:53.3", "23:53.4", "23:53.4", "23:53.4", "23:53.5", "23:53.5", "23:53.5", "23:53.6", "23:53.6", "23:53.6", "23:53.7", "23:53.7", "23:53.7", "23:53.8", "23:53.8", "23:53.8", "23:53.9", "23:53.9", "23:53.9", "23:54.0", "23:54.0", "23:54.0", "23:54.1", "23:54.1", "23:54.1", "23:54.2", "23:54.2", "23:54.2", "23:54.3", "23:54.3", "23:54.3", "23:54.4", "23:54.4", "23:54.4", "23:54.5", "23:54.5", "23:54.5", "23:54.6", "23:54.6", "23:54.6", "23:54.7", "23:54.7", "23:54.7", "23:54.8", "23:54.8", "23:54.8", "23:54.9", "23:54.9", "23:54.9", "23:55.0", "23:55.0", "23:55.0", "23:55.1", "23:55.1", "23:55.1", "23:55.2", "23:55.2", "23:55.2", "23:55.3", "23:55.3", "23:55.3", "23:55.4", "23:55.4", "23:55.4", "23:55.5", "23:55.5", "23:55.5", "23:55.6", "23:55.6", "23:55.6", "23:55.7", "23:55.7", "23:55.7", "23:55.8", "23:55.8", "23:55.8", "23:55.9", "23:55.9", "23:55.9", "23:56.0", "23:56.0", "23:56.0", "23:56.1", "23:56.1", "23:56.1", "23:56.2", "23:56.2", "23:56.2", "23:56.3", "23:56.3", "23:56.3", "23:56.4", "23:56.4", "23:56.4", "23:56.5", "23:56.5", "23:56.5", "23:56.6", "23:56.6", "23:56.6", "23:56.7", "23:56.7", "23:56.7", "23:56.8", "23:56.8", "23:56.8", "23:56.9", "23:56.9", "23:56.9", "23:57.0", "23:57.0", "23:57.0", "23:57.1", "23:57.1", "23:57.1", "23:57.2", "23:57.2", "23:57.2", "23:57.3", "23:57.3", "23:57.3", "23:57.4", "23:57.4", "23:57.4", "23:57.5", "23:57.5", "23:57.5", "23:57.6", "23:57.6", "23:57.6", "23:57.7", "23:57.7", "23:57.7", "23:57.8", "23:57.8", "23:57.8", "23:57.9", "23:57.9", "23:57.9", "23:58.0", "23:58.0", "23:58.0", "23:58.1", "23:58.1", "23:58.1", "23:58.2", "23:58.2", "23:58.2", "23:58.3", "23:58.3", "23:58.3", "23:58.4", "23:58.4", "23:58.4", "23:58.5", "23:58.5", "23:58.5", "23:58.6", "23:58.6", "23:58.6", "23:58.7", "23:58.7", "23:58.7", "23:58.8", "23:58.8", "23:58.8", "23:58.9", "23:58.9", "23:58.9", "23:59.0", "23:59.0", "23:59.0", "23:59.1", "23:59.1", "23:59.1", "23:59.2", "23:59.2", "23:59.2", "23:59.3", "23:59.3", "23:59.3", "23:59.4", "23:59.4", "23:59.4", "23:59.5", "23:59.5", "23:59.5", "23:59.6", "23:59.6", "23:59.6", "23:59.7", "23:59.7", "23:59.7", "23:59.8", "23:59.8", "23:59.8", "23:59.9", "23:59.9", "23:59.9", "24:00.0", "24:00.0", "24:00.0", "24:00.1", "24:00.1", "24:00.1", "24:00.2", "24:00.2", "24:00.2", "24:00.3", "24:00.3", "24:00.3", "24:00.4", "24:00.4", "24:00.4", "24:00.5", "24:00.5", "24:00.5", "24:00.6", "24:00.6", "24:00.6", "24:00.7", "24:00.7", "24:00.7", "24:00.8", "24:00.8", "24:00.8", "24:00.9", "24:00.9", "24:00.9", "24:01.0", "24:01.0", "24:01.0", "24:01.1", "24:01.1", "24:01.1", "24:01.2", "24:01.2", "24:01.2", "24:01.3", "24:01.3", "24:01.3", "24:01.4", "24:01.4", "24:01.4", "24:01.5", "24:01.5", "24:01.5", "24:01.6", "24:01.6", "24:01.6", "24:01.7", "24:01.7", "24:01.7", "24:01.8", "24:01.8", "24:01.8", "24:01.9", "24:01.9", "24:01.9", "24:02.0", "24:02.0", "24:02.0", "24:02.1", "24:02.1", "24:02.1", "24:02.2", "24:02.2", "24:02.2", "24:02.3", "24:02.3", "24:02.3", "24:02.4", "24:02.4", "24:02.4", "24:02.5", "24:02.5", "24:02.5", "24:02.6", "24:02.6", "24:02.6", "24:02.7", "24:02.7", "24:02.7", "24:02.8", "24:02.8", "24:02.8", "24:02.9", "24:02.9", "24:02.9", "24:03.0", "24:03.0", "24:03.0", "24:03.1", "24:03.1", "24:03.1", "24:03.2", "24:03.2", "24:03.2", "24:03.3", "24:03.3", "24:03.3", "24:03.4", "24:03.4", "24:03.4", "24:03.5", "24:03.5", "24:03.5", "24:03.6", "24:03.6", "24:03.6", "24:03.7", "24:03.7", "24:03.7", "24:03.8", "24:03.8", "24:03.8", "24:03.9", "24:03.9", "24:03.9", "24:04.0", "24:04.0", "24:04.0", "24:04.1", "24:04.1", "24:04.1", "24:04.2", "24:04.2", "24:04.2", "24:04.3", "24:04.3", "24:04.3", "24:04.4", "24:04.4", "24:04.4", "24:04.5", "24:04.5", "24:04.5", "24:04.6", "24:04.6", "24:04.6", "24:04.7", "24:04.7", "24:04.7", "24:04.8", "24:04.8", "24:04.8", "24:04.9", "24:04.9", "24:04.9", "24:05.0", "24:05.0", "24:05.0", "24:05.1", "24:05.1", "24:05.1", "24:05.2", "24:05.2", "24:05.2", "24:05.3", "24:05.3", "24:05.3", "24:05.4", "24:05.4", "24:05.4", "24:05.5", "24:05.5", "24:05.5", "24:05.6", "24:05.6", "24:05.6", "24:05.7", "24:05.7", "24:05.7", "24:05.8", "24:05.8", "24:05.8", "24:05.9", "24:05.9", "24:05.9", "24:06.0", "24:06.0", "24:06.0", "24:06.1", "24:06.1", "24:06.1", "24:06.2", "24:06.2", "24:06.2", "24:06.3", "24:06.3", "24:06.3", "24:06.4", "24:06.4", "24:06.4", "24:06.5", "24:06.5", "24:06.5", "24:06.6", "24:06.6", "24:06.6", "24:06.7", "24:06.7", "24:06.7", "24:06.8", "24:06.8", "24:06.8", "24:06.9", "24:06.9", "24:06.9", "24:07.0", "24:07.0", "24:07.0", "24:07.1", "24:07.1", "24:07.1", "24:07.2", "24:07.2", "24:07.2", "24:07.3", "24:07.3", "24:07.3", "24:07.4", "24:07.4", "24:07.4", "24:07.5", "24:07.5", "24:07.5", "24:07.6", "24:07.6", "24:07.6", "24:07.7", "24:07.7", "24:07.7", "24:07.8", "24:07.8", "24:07.8", "24:07.9", "24:07.9", "24:07.9", "24:08.0", "24:08.0", "24:08.0", "24:08.1", "24:08.1", "24:08.1", "24:08.2", "24:08.2", "24:08.2", "24:08.3", "24:08.3", "24:08.3", "24:08.4", "24:08.4", "24:08.4", "24:08.5", "24:08.5", "24:08.5", "24:08.6", "24:08.6", "24:08.6", "24:08.7", "24:08.7", "24:08.7", "24:08.8", "24:08.8", "24:08.8", "24:08.9", "24:08.9", "24:08.9", "24:09.0", "24:09.0", "24:09.0", "24:09.1", "24:09.1", "24:09.1", "24:09.2", "24:09.2", "24:09.2", "24:09.3", "24:09.3", "24:09.3", "24:09.4", "24:09.4", "24:09.4", "24:09.5", "24:09.5", "24:09.5", "24:09.6", "24:09.6", "24:09.6", "24:09.7", "24:09.7", "24:09.7", "24:09.8", "24:09.8", "24:09.8", "24:09.9", "24:09.9", "24:09.9", "24:10.0", "24:10.0", "24:10.0", "24:10.1", "24:10.1", "24:10.1", "24:10.2", "24:10.2", "24:10.2", "24:10.3", "24:10.3", "24:10.3", "24:10.4", "24:10.4", "24:10.4", "24:10.5", "24:10.5", "24:10.5", "24:10.6", "24:10.6", "24:10.6", "24:10.7", "24:10.7", "24:10.7", "24:10.8", "24:10.8", "24:10.8", "24:10.9", "24:10.9", "24:10.9", "24:11.0", "24:11.0", "24:11.0", "24:11.1", "24:11.1", "24:11.1", "24:11.2", "24:11.2", "24:11.2", "24:11.3", "24:11.3", "24:11.3", "24:11.4", "24:11.4", "24:11.4", "24:11.5", "24:11.5", "24:11.5", "24:11.6", "24:11.6", "24:11.6", "24:11.7", "24:11.7", "24:11.7", "24:11.8", "24:11.8", "24:11.8", "24:11.9", "24:11.9", "24:11.9", "24:12.0", "24:12.0", "24:12.0", "24:12.1", "24:12.1", "24:12.1", "24:12.2", "24:12.2", "24:12.2", "24:12.3", "24:12.3", "24:12.3", "24:12.4", "24:12.4", "24:12.4", "24:12.5", "24:12.5", "24:12.5", "24:12.6", "24:12.6", "24:12.6", "24:12.7", "24:12.7", "24:12.7", "24:12.8", "24:12.8", "24:12.8", "24:12.9", "24:12.9", "24:12.9", "24:13.0", "24:13.0", "24:13.0", "24:13.1", "24:13.1", "24:13.1", "24:13.2", "24:13.2", "24:13.2", "24:13.3", "24:13.3", "24:13.3", "24:13.4", "24:13.4", "24:13.4", "24:13.5", "24:13.5", "24:13.5", "24:13.6", "24:13.6", "24:13.6", "24:13.7", "24:13.7", "24:13.7", "24:13.8", "24:13.8", "24:13.8", "24:13.9", "24:13.9", "24:13.9", "24:14.0", "24:14.0", "24:14.0", "24:14.1", "24:14.1", "24:14.1", "24:14.2", "24:14.2", "24:14.2", "24:14.3", "24:14.3", "24:14.3", "24:14.4", "24:14.4", "24:14.4", "24:14.5", "24:14.5", "24:14.5", "24:14.6", "24:14.6", "24:14.6", "24:14.7", "24:14.7", "24:14.7", "24:14.8", "24:14.8", "24:14.8", "24:14.9", "24:14.9", "24:14.9", "24:15.0", "24:15.0", "24:15.0", "24:15.1", "24:15.1", "24:15.1", "24:15.2", "24:15.2", "24:15.2", "24:15.3", "24:15.3", "24:15.3", "24:15.4", "24:15.4", "24:15.4", "24:15.5", "24:15.5", "24:15.5", "24:15.6", "24:15.6", "24:15.6", "24:15.7", "24:15.7", "24:15.7", "24:15.8", "24:15.8", "24:15.8", "24:15.9", "24:15.9", "24:15.9", "24:16.0", "24:16.0", "24:16.0", "24:16.1", "24:16.1", "24:16.1", "24:16.2", "24:16.2", "24:16.2", "24:16.3", "24:16.3", "24:16.3", "24:16.4", "24:16.4", "24:16.4", "24:16.5", "24:16.5", "24:16.5", "24:16.6", "24:16.6", "24:16.6", "24:16.7", "24:16.7", "24:16.7", "24:16.8", "24:16.8", "24:16.8", "24:16.9", "24:16.9", "24:16.9", "24:17.0", "24:17.0", "24:17.0", "24:17.1", "24:17.1", "24:17.1", "24:17.2", "24:17.2", "24:17.2", "24:17.3", "24:17.3", "24:17.3", "24:17.4", "24:17.4", "24:17.4", "24:17.5", "24:17.5", "24:17.5", "24:17.6", "24:17.6", "24:17.6", "24:17.7", "24:17.7", "24:17.7", "24:17.8", "24:17.8", "24:17.8", "24:17.9", "24:17.9", "24:17.9", "24:18.0", "24:18.0", "24:18.0", "24:18.1", "24:18.1", "24:18.1", "24:18.2", "24:18.2", "24:18.2", "24:18.3", "24:18.3", "24:18.3", "24:18.4", "24:18.4", "24:18.4", "24:18.5", "24:18.5", "24:18.5", "24:18.6", "24:18.6", "24:18.6", "24:18.7", "24:18.7", "24:18.7", "24:18.8", "24:18.8", "24:18.8", "24:18.9", "24:18.9", "24:18.9", "24:19.0", "24:19.0", "24:19.0", "24:19.1", "24:19.1", "24:19.1", "24:19.2", "24:19.2", "24:19.2", "24:19.3", "24:19.3", "24:19.3", "24:19.4", "24:19.4", "24:19.4", "24:19.5", "24:19.5", "24:19.5", "24:19.6", "24:19.6", "24:19.6", "24:19.7", "24:19.7", "24:19.7", "24:19.8", "24:19.8", "24:19.8", "24:19.9", "24:19.9", "24:19.9", "24:20.0", "24:20.0", "24:20.0", "24:20.1", "24:20.1", "24:20.1", "24:20.2", "24:20.2", "24:20.2", "24:20.3", "24:20.3", "24:20.3", "24:20.4", "24:20.4", "24:20.4", "24:20.5", "24:20.5", "24:20.5", "24:20.6", "24:20.6", "24:20.6", "24:20.7", "24:20.7", "24:20.7", "24:20.8", "24:20.8", "24:20.8", "24:20.9", "24:20.9", "24:20.9", "24:21.0", "24:21.0", "24:21.0", "24:21.1", "24:21.1", "24:21.1", "24:21.2", "24:21.2", "24:21.2", "24:21.3", "24:21.3", "24:21.3", "24:21.4", "24:21.4", "24:21.4", "24:21.5", "24:21.5", "24:21.5", "24:21.6", "24:21.6", "24:21.6", "24:21.7", "24:21.7", "24:21.7", "24:21.8", "24:21.8", "24:21.8", "24:21.9", "24:21.9", "24:21.9", "24:22.0", "24:22.0", "24:22.0", "24:22.1", "24:22.1", "24:22.1", "24:22.2", "24:22.2", "24:22.2", "24:22.3", "24:22.3", "24:22.3", "24:22.4", "24:22.4", "24:22.4", "24:22.5", "24:22.5", "24:22.5", "24:22.6", "24:22.6", "24:22.6", "24:22.7", "24:22.7", "24:22.7", "24:22.8", "24:22.8", "24:22.8", "24:22.9", "24:22.9", "24:22.9", "24:23.0", "24:23.0", "24:23.0", "24:23.1", "24:23.1", "24:23.1", "24:23.2", "24:23.2", "24:23.2", "24:23.3", "24:23.3", "24:23.3", "24:23.4", "24:23.4", "24:23.4", "24:23.5", "24:23.5", "24:23.5", "24:23.6", "24:23.6", "24:23.6", "24:23.7", "24:23.7", "24:23.7", "24:23.8", "24:23.8", "24:23.8", "24:23.9", "24:23.9", "24:23.9", "24:24.0", "24:24.0", "24:24.0", "24:24.1", "24:24.1", "24:24.1", "24:24.2", "24:24.2", "24:24.2", "24:24.3", "24:24.3", "24:24.3", "24:24.4", "24:24.4", "24:24.4", "24:24.5", "24:24.5", "24:24.5", "24:24.6", "24:24.6", "24:24.6", "24:24.7", "24:24.7", "24:24.7", "24:24.8", "24:24.8", "24:24.8", "24:24.9", "24:24.9", "24:24.9", "24:25.0", "24:25.0", "24:25.0", "24:25.1", "24:25.1", "24:25.1", "24:25.2", "24:25.2", "24:25.2", "24:25.3", "24:25.3", "24:25.3", "24:25.4", "24:25.4", "24:25.4", "24:25.5", "24:25.5", "24:25.5", "24:25.6", "24:25.6", "24:25.6", "24:25.7", "24:25.7", "24:25.7", "24:25.8", "24:25.8", "24:25.8", "24:25.9", "24:25.9", "24:25.9", "24:26.0", "24:26.0", "24:26.0", "24:26.1", "24:26.1", "24:26.1", "24:26.2", "24:26.2", "24:26.2", "24:26.3", "24:26.3", "24:26.3", "24:26.4", "24:26.4", "24:26.4", "24:26.5", "24:26.5", "24:26.5", "24:26.6", "24:26.6", "24:26.6", "24:26.7", "24:26.7", "24:26.7", "24:26.8", "24:26.8", "24:26.8", "24:26.9", "24:26.9", "24:26.9", "24:27.0", "24:27.0", "24:27.0", "24:27.1", "24:27.1", "24:27.1", "24:27.2", "24:27.2", "24:27.2", "24:27.3", "24:27.3", "24:27.3", "24:27.4", "24:27.4", "24:27.4", "24:27.5", "24:27.5", "24:27.5", "24:27.6", "24:27.6", "24:27.6", "24:27.7", "24:27.7", "24:27.7", "24:27.8", "24:27.8", "24:27.8", "24:27.9", "24:27.9", "24:27.9", "24:28.0", "24:28.0", "24:28.0", "24:28.1", "24:28.1", "24:28.1", "24:28.2", "24:28.2", "24:28.2", "24:28.3", "24:28.3", "24:28.3", "24:28.4", "24:28.4", "24:28.4", "24:28.5", "24:28.5", "24:28.5", "24:28.6", "24:28.6", "24:28.6", "24:28.7", "24:28.7", "24:28.7", "24:28.8", "24:28.8", "24:28.8", "24:28.9", "24:28.9", "24:28.9", "24:29.0", "24:29.0", "24:29.0", "24:29.1", "24:29.1", "24:29.1", "24:29.2", "24:29.2", "24:29.2", "24:29.3", "24:29.3", "24:29.3", "24:29.4", "24:29.4", "24:29.4", "24:29.5", "24:29.5", "24:29.5", "24:29.6", "24:29.6", "24:29.6", "24:29.7", "24:29.7", "24:29.7", "24:29.8", "24:29.8", "24:29.8", "24:29.9", "24:29.9", "24:29.9", "24:30.0", "24:30.0", "24:30.0", "24:30.1", "24:30.1", "24:30.1", "24:30.2", "24:30.2", "24:30.2", "24:30.3", "24:30.3", "24:30.3", "24:30.4", "24:30.4", "24:30.4", "24:30.5", "24:30.5", "24:30.5", "24:30.6", "24:30.6", "24:30.6", "24:30.7", "24:30.7", "24:30.7", "24:30.8", "24:30.8", "24:30.8", "24:30.9", "24:30.9", "24:30.9", "24:31.0", "24:31.0", "24:31.0", "24:31.1", "24:31.1", "24:31.1", "24:31.2", "24:31.2", "24:31.2", "24:31.3", "24:31.3", "24:31.3", "24:31.4", "24:31.4", "24:31.4", "24:31.5", "24:31.5", "24:31.5", "24:31.6", "24:31.6", "24:31.6", "24:31.7", "24:31.7", "24:31.7", "24:31.8", "24:31.8", "24:31.8", "24:31.9", "24:31.9", "24:31.9", "24:32.0", "24:32.0", "24:32.0", "24:32.1", "24:32.1", "24:32.1", "24:32.2", "24:32.2", "24:32.2", "24:32.3", "24:32.3", "24:32.3", "24:32.4", "24:32.4", "24:32.4", "24:32.5", "24:32.5", "24:32.5", "24:32.6", "24:32.6", "24:32.6", "24:32.7", "24:32.7", "24:32.7", "24:32.8", "24:32.8", "24:32.8", "24:32.9", "24:32.9", "24:32.9", "24:33.0", "24:33.0", "24:33.0", "24:33.1", "24:33.1", "24:33.1", "24:33.2", "24:33.2", "24:33.2", "24:33.3", "24:33.3", "24:33.3", "24:33.4", "24:33.4", "24:33.4", "24:33.5", "24:33.5", "24:33.5", "24:33.6", "24:33.6", "24:33.6", "24:33.7", "24:33.7", "24:33.7", "24:33.8", "24:33.8", "24:33.8", "24:33.9", "24:33.9", "24:33.9", "24:34.0", "24:34.0", "24:34.0", "24:34.1", "24:34.1", "24:34.1", "24:34.2", "24:34.2", "24:34.2", "24:34.3", "24:34.3", "24:34.3", "24:34.4", "24:34.4", "24:34.4", "24:34.5", "24:34.5", "24:34.5", "24:34.6", "24:34.6", "24:34.6", "24:34.7", "24:34.7", "24:34.7", "24:34.8", "24:34.8", "24:34.8", "24:34.9", "24:34.9", "24:34.9", "24:35.0", "24:35.0", "24:35.0", "24:35.1", "24:35.1", "24:35.1", "24:35.2", "24:35.2", "24:35.2", "24:35.3", "24:35.3", "24:35.3", "24:35.4", "24:35.4", "24:35.4", "24:35.5", "24:35.5", "24:35.5", "24:35.6", "24:35.6", "24:35.6", "24:35.7", "24:35.7", "24:35.7", "24:35.8", "24:35.8", "24:35.8", "24:35.9", "24:35.9", "24:35.9", "24:36.0", "24:36.0", "24:36.0", "24:36.1", "24:36.1", "24:36.1", "24:36.2", "24:36.2", "24:36.2", "24:36.3", "24:36.3", "24:36.3", "24:36.4", "24:36.4", "24:36.4", "24:36.5", "24:36.5", "24:36.5", "24:36.6", "24:36.6", "24:36.6", "24:36.7", "24:36.7", "24:36.7", "24:36.8", "24:36.8", "24:36.8", "24:36.9", "24:36.9", "24:36.9", "24:37.0", "24:37.0", "24:37.0", "24:37.1", "24:37.1", "24:37.1", "24:37.2", "24:37.2", "24:37.2", "24:37.3", 
